vi "Lookup Global Channels.vi"(8 "error in (no error)":errorcluster, 11 "Item Ref in":T2 format="%.0x") -> (0 "error out":errorcluster, 2 "Channel Lookup Info":T1 {"Refs" format="%.0x"}, 3 "Section Ref out":T2 format="%.0x")   [LabVIEW 2019, in "Instrument Addon System Explorer.lvlib"]
uses:
  Instrument Addon System Explorer.lvlib
  <vilib>/NI VeriStand/Custom Device API/Custom Device Item Ref.ctl
  Types/Channel Lookup Cluster.ctl
  Addon Shared/SubVIs/MetaData Parameters FG.vi
  Addon Shared/SubVIs/Constants.vi
  <vilib>/NI VeriStand/Custom Device Tools/Custom Device Utility Library/NI VeriStand - Search for Item by GUID.vi
  <vilib>/NI VeriStand/Custom Device API/NI VeriStand - Get Item Property.vi
  <vilib>/NI VeriStand/Custom Device API/Get Item Property (U32).vi
  <vilib>/NI VeriStand/Custom Device API/Get Item Property (String Array).vi
  <vilib>/NI VeriStand/Custom Device API/Get Item Property (String).vi
  <vilib>/NI VeriStand/Custom Device API/NI VeriStand - Set Item Property.vi
  <vilib>/NI VeriStand/Custom Device API/Set Item Property (U32).vi
  <vilib>/NI VeriStand/Custom Device API/Set Item Property (String Array).vi
  <vilib>/NI VeriStand/Custom Device API/NI VeriStand - Set Custom Device Channel Value Table.vi
  <vilib>/NI VeriStand/Custom Device API/Set Item Property (String).vi
  <vilib>/NI VeriStand/Custom Device Tools/Custom Device Utility Library/Custom Device Utility Library.lvlib
  Addon Shared/Instrument Addon Shared.lvlib
  <vilib>/NI VeriStand/Custom Device API/Custom Device API.lvlib
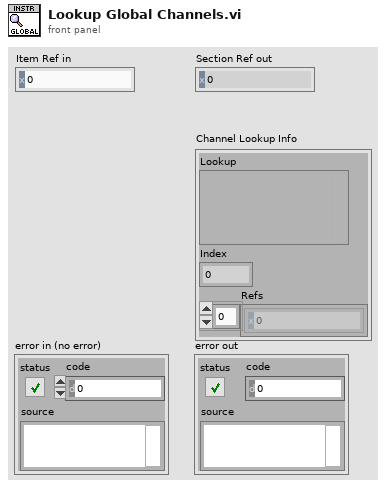
[diagram p1: front panel]
types:
  T1 = typedef "Instrument Addon System Explorer.lvlib/Channel Lookup Cluster.ctl" = cluster{"Lookup":variant, "Index":i32, "Refs":T2[]}
  T2 = typedef "Custom Device API.lvlib/Custom Device Item Ref.ctl" = u64
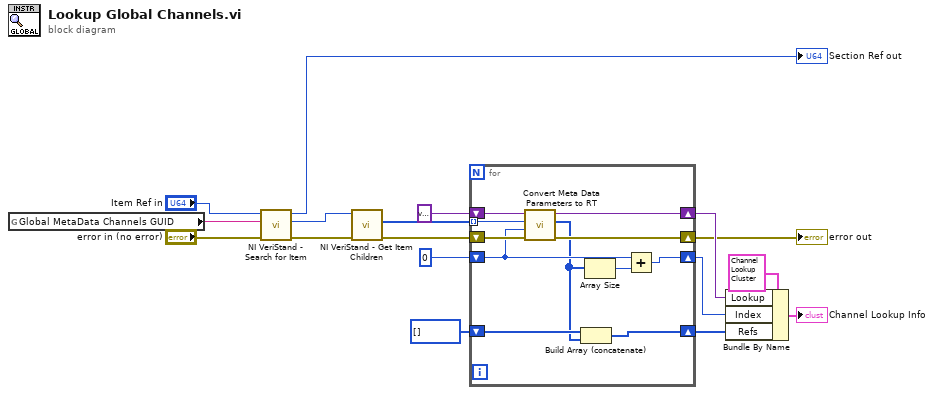
[diagram p0: block diagram]
diagram:
  n1 = global read "Constants.vi" "Global MetaData Channels GUID"() -> (w12:string)
  n2 = call-poly <vilib>:"NI VeriStand - Search for Item.vi"("error in"="error in (no error)", "Item GUID"=w12, "Section Ref in"="Item Ref in") -> ("error out"=w14:errorcluster, "Item Ref"=w13:T2, "Section Ref out"=→"Section Ref out":T2)  [unwired: 5 in, 1 out]
  n3 = call <vilib>:"NI VeriStand - Get Item Children.vi"("error in (no error)"=w14, "Item Ref in"=w13) -> ("error out"=w6:errorcluster, "Child Refs"=w7:T2[])  [unwired: 6 in, 2 out]
  n4 = for {
    shift-right: [w23] -> w2
    shift-left: w6 -> [w27]
    tunnel: w7 -> [w26] mode=indexing
    shift-right: [w28] -> w9
    shift-left: 0 -> [w21]
    shift-right: [w24] -> w3
    shift-left: variant ("variant") -> [w25]
    shift-right: [w19] -> w8
    shift-left: T2[] [] -> [w20]
    n5 = call "Convert Meta Data Parameters to RT.vi"("error in (no error)"=w27, "Data Index"=w21, "Item Ref in"=w26, "Lookup Table"=w25) -> ("error out"=w23:errorcluster, "Chan Refs"=w18:T2[], "Lookup Table out"=w24:variant)  [unwired: 5 in]
    n6 = Build Array (concatenate)(w20, w18) -> (w19:T2[])
    n7 = Array Size(array=w18) -> (size(s)=w22:i32)
    n8 = Add(x=w21, y=w22) -> (x+y=w28:i32)
  }
  "error out" <- w2
  n9 = Bundle By Name(cluster=T1 {"Lookup"=variant, "Index"=0, "Refs"=[]}, "Lookup"=w3, "Index"=w9, "Refs"=w8) -> (→"Channel Lookup Info":T1)
